vi "Time_DataTime String To Time Stamp.vi"(8 "Time Split(:)":string=":", 9 "Date Split(/)":string="/", 10 "Split( )":string=" ", 11 "DataTime String":string) -> (3 "Time Stamp":timestamp)   [LabVIEW 2016]
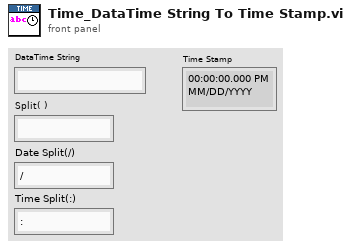
[diagram p1: front panel]
types:
  T1 = typedef "LVDateTimeRec.ctl" = cluster{"秒数的小数部分":dbl, "秒":i32, "分":i32, "时":i32, "日":i32, "月":i32, "年":i32, "天数（周）":i32, "天数（年）":i32, "DST":i32}
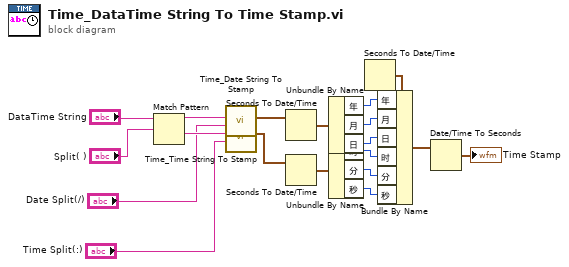
[diagram p0: block diagram]
diagram:
  n1 = Match Pattern(string="DataTime String", regular expression="Split( )") -> (before substring=w18:string, after substring=w17:string)  [unwired: 1 in, 2 out]
  n2 = call "Time_Date String To Stamp.vi"("Split"="Date Split(/)", "Data String"=w18) -> ("Time Stamp"=w15:timestamp)  [unwired: 9 in]
  n3 = call "Time_Time String To Stamp.vi"("Split"="Time Split(:)", "Data String"=w17) -> ("Time Stamp"=w10:timestamp)  [unwired: 9 in]
  n4 = Seconds To Date/Time(time stamp (now)=w15) -> (date time rec=w14:T1)  [unwired: 1 in]
  n5 = Seconds To Date/Time(time stamp (now)=w10) -> (date time rec=w8:T1)  [unwired: 1 in]
  n6 = Unbundle By Name(w14) -> ("年"=w13:i32, "月"=w12:i32, "日"=w11:i32)
  n7 = Unbundle By Name(w8) -> ("时"=w9:i32, "分"=w7:i32, "秒"=w6:i32)
  n8 = Seconds To Date/Time() -> (date time rec=w16:T1)  [unwired: 2 in]
  n9 = Bundle By Name(cluster=w16, "年"=w13, "月"=w12, "日"=w11, "时"=w9, "分"=w7, "秒"=w6) -> (w5:T1)
  n10 = Date/Time To Seconds(2:w5) -> (0:→"Time Stamp":timestamp)  [unwired: 1 in]
